vi "Auto Intake Mode.vi"(7 "Intake Angle":dbl, 11 "Intake Commands Cluster":T2={"Intake Commands"=enum."Load", "Intake Mode"=enum."Auto", "Override IR"=FALSE, "Angle Target"=0.0}) -> (0 "Intake States":T1, 1 "Limit with Encoders?":bool, 2 "Roller Power":dbl, 3 "Angle Power":dbl, 4 "Target Height":dbl, 5 "Encoder Position":dbl, 6 "Rollers Active?":bool)   [LabVIEW 2015]
uses:
  Common Code/Intake Commands Cluster.ctl
  Common Code/Intake Commands.ctl
  Common Code/Intake Mode.ctl
  Common Code/Intake States.ctl
  Common Code/Change Detect Int.vi
  Common Code/Change Detect Double.vi
  Robot Global Data.vi
  <vilib>/addons/control/pid/pid.llb/PID (DBL).vi
  <vilib>/addons/control/pid/NI_PID_pid.lvlib
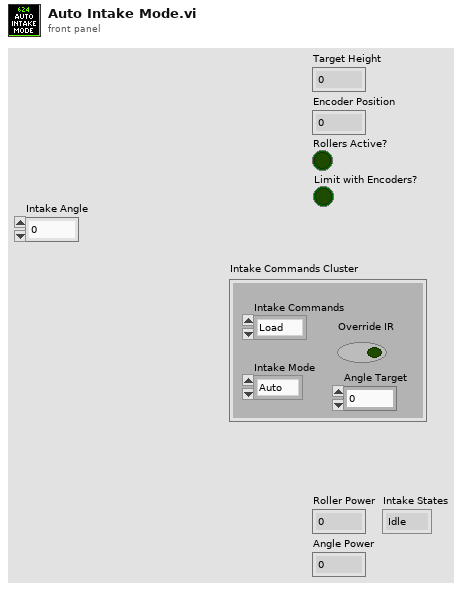
[diagram p1: front panel]
types:
  T1 = typedef "Intake States.ctl" = enum16{"Idle", "Set roller speed", "Move to angle", "Go Hard or Go Home", "Ball Settle"}
  T2 = typedef "Intake Commands Cluster.ctl" = cluster{"Intake Commands":T3, "Intake Mode":T4, "Override IR":bool, "Angle Target":dbl}
  T3 = typedef "Intake Commands.ctl" = enum16{"Settle Ball", "Unload", "Load", "Pull up", "Drop low", "Idle", "Lift Half", "Go To Angle"}
  T4 = typedef "Intake Mode.ctl" = enum16{"Safe", "Auto", "Manual"}
  T5 = typedef "Dashboard Control Data.ctl" = cluster{"Shooter Presets":T6, "Encoder Control":T8, "Steer PID output":cluster{"output high":dbl, "output low":dbl}, " Steer PID gains":cluster{"proportional gain (Kc)":dbl, "integral time (Ti, min)":dbl, "derivative time (Td, min)":dbl}, "Drivetrain Settings":T9, "Vision Packet":T10, "Dashboard Drivetrain Command":T11, "Info/Command Cluster":T13, "Ball Vision Packet":T14, "Intake Presets":T16, "Intake Encoder Control":T18, "Climb Presets":T19, "Goal Output Range":cluster{"output high":dbl, "output low":dbl}, "Enabled Systems":T20, "Auton Presets":T21, "Pressure M":dbl, "Pressure B":dbl, "Vision Timeout":dbl, "Auto-Shift":T22}
  T6 = typedef "Shooter Presets.ctl" = cluster{"Batter Shot":T7, "Deep Middle":T7, "Manual Shot":T7, "Left Ticks Per Rotation":dbl, "Right Ticks Per Rotation":dbl, "Low Bar Shot":T7, "Shooter RPM Tolerance":dbl, "Trigger Power":dbl, "Fire from Load Delay":i32, "Max Angle":dbl, "Min Angle":dbl, "Angle PID gains":cluster{"P":dbl, "I":dbl, "D":dbl}, "Angle Output":cluster{"output high":dbl, "output low":dbl}, "Shooter Angle Tolerance":dbl, "Vision Shoot x^2":dbl, "Vision Shoot x":dbl, "Feed Forward Max Accel":dbl, "Feed Forward Kv":dbl, "Backwards Trigger":dbl, "Shot Finish Delay (ms)":dbl, "Angle Max Current":dbl, "Angle Current Trip Time":dbl, "Intake Angle":dbl, "Vision Shoot c":dbl, "Reset?":bool, "Button Release Delay":dbl, "Angle Pot x":dbl, "Angle Pot c":dbl, "Ignore Angle?":bool, "Max RPM":dbl, "Safty Frist Angle":dbl, "Intake Danger Height":dbl, "Angle Pot B":i32, "Angle Pot M":dbl, "FF Finish RPM":dbl, "RPM PID Right":cluster{"P":dbl, "I":dbl, "D":dbl, "FF":dbl}, "RPM PID Left":cluster{"P":dbl, "I":dbl, "D":dbl, "FF":dbl}, "Backwards RPM":dbl, "Vision RPM":dbl, "Run Wheels Backward Delay":u32, "Cleat Shot":T7}
  T7 = typedef "Shot Presets.ctl" = cluster{"L":dbl, "R":dbl, "A":dbl}
  T8 = typedef "Encoder Control.ctl" = cluster{"Right Tick Constant":dbl, "Left Tick Constant":dbl, "Reset?":bool, "Y Dist":cluster{"PID gains":cluster{"proportional gain (Kc)":dbl, "integral time (Ti, min)":dbl, "derivative time (Td, min)":dbl}}, "Y Stop Thresh":dbl, "Y Stop Speed":dbl}
  T9 = typedef "Drivetrain Settings.ctl" = cluster{"Gyro Tolerance":dbl, "Throttle Ramp (ms)":dbl, "Kv":dbl, "Ka":dbl, "Feed Forward P":dbl, "Feed Forward D":dbl, "Goal Vision PID gains":cluster{"proportional gain (Kc)":dbl, "integral time (Ti, min)":dbl, "derivative time (Td, min)":dbl}, "Goal Detection Window":dbl, "Creep Rate":dbl, "Vision Throttle Threshold":dbl, "Min Turn Output":dbl, "Left Batter Angle":dbl, "Right Batter Angle":dbl}
  T10 = typedef "Goal Vision Packet.ctl" = cluster{"Distance":dbl, "Center X":dbl, "Center Y":dbl, "Found Target?":bool, "Robot Center":dbl, "Angle":dbl}
  T11 = typedef "Dashboard Drivetrain Command.ctl" = cluster{"Drivetrain Vision":T12}
  T12 = typedef "Drivetrain Vision.ctl" = cluster{"Goal Window":dbl, "Ball Window":dbl}
  T13 = typedef "Ball Tracking Command Cluster.ctl" = cluster{"Distance to Ball":dbl, "Desired Angle":dbl, "Command":enum16{"Turn to Ball", "Turn to Angle", "Get Distance"}, "Pixels from Center":dbl}
  T14 = typedef "Ball Vision Packet.ctl" = cluster{"Ball Detected?":bool, "Distance to Ball":dbl, "Desired Angle":dbl, "Pixels from Center":dbl, "Tracking mode":T15}
  T15 = typedef "Tracking Mode.ctl" = enum16{"Turn to Ball", "Turn to Angle"}
  T16 = typedef "Intake Presets.ctl" = cluster{"Intake Speed":dbl, "Outake Speed":dbl, "Low Height":dbl, "Half Height":dbl, "High Idle Height":dbl, "Angle Speed":dbl, "Angle Tolerance":dbl, "Encoder Scale":dbl, "Load Height":dbl, "Output Range":T17, "Rotation Power Max/Min":dbl, "MaxCurrent":dbl, "Intake Trip Time":dbl, "Idle Height":dbl, "Max Height":dbl, "Reset Encoders?":bool, "PID gains":cluster{"proportional gain (Kc)":dbl, "integral time (Ti, min)":dbl, "derivative time (Td, min)":dbl}, "Intake Stop Delay":u32, "Settle Time":dbl, "Settle Wait Time":dbl, "Pull Up Delay":dbl}
  T17 = typedef "Drivetrain Output Range.ctl" = cluster{"output high":dbl, "output low":dbl}
  T18 = typedef "IntakeEcoderControl.ctl" = cluster{"Arm Tick Constant":dbl, "Reset?":bool, "Y Dist":cluster{"PID gains":cluster{"proportional gain (Kc)":dbl, "integral time (Ti, min)":dbl, "derivative time (Td, min)":dbl}}, "Y Stop Thresh":dbl, "Y Stop Speed":dbl}
  T19 = typedef "Climb Presets.ctl" = cluster{"Pull Power":dbl, "Extend Power":dbl}
  T20 = typedef "Enabled Systems.ctl" = cluster{"Shoot":bool, "Intake":bool, "DT":bool, "Gyro":bool, "100ms":bool, "US":bool}
  T21 = typedef "Autonomous Presets.ctl" = cluster{"Pitch Limit":dbl, "Roll Limit":dbl, "Start Position":dbl, "Cross Position":dbl}
  T22 = typedef "Auto Shift Cluster.ctl" = cluster{"Delay":dbl, "Speed Thresh":dbl, "Upshift Accel":dbl, "Upshift Throttle":dbl, "Upshift Throttle Accel":dbl, "Downshift Throttle":dbl, "Downshift Throttle Accel":dbl}
  T23 = cluster{"proportional gain (Kc)":dbl, "integral time (Ti, min)":dbl, "derivative time (Td, min)":dbl}
  T24 = typedef "Shooter State Cluster.ctl" = cluster{"State":T25, "Left RPM":dbl, "Right RPM":dbl, "Shooter Ready?":bool, "Ball Loaded?":bool, "Current Angle":dbl, "Angle Motor Output":dbl, "Trigger Output":dbl, "Angle Ready?":bool, "RPM Ready?":bool, "Vision Ready?":bool, "Ball Loaded?":bool, "Mode":T26, "Shot Type":T27, "Pot Height":dbl, "Current Tripped Forward?":bool, "Current Tripped Backward?":bool, "Right Servo":i32, "Left Servo":i32, "IR Override":bool, "Intake Danger?":bool, "Intake Angle Ready?":bool}
  T25 = typedef "Shooter State.ctl" = enum16{"Idle", "Settle Ball", "Warmup", "Shooter Ready", "Shoot"}
  T26 = typedef "Shoot Modes Enum.ctl" = enum16{"Manual", "Safe", "Auto"}
  T27 = typedef "Shot Type.ctl" = enum16{"Batter Shot", "Corner Shot", "Cleat Shot", "Vision Shot", "Deep Middle Shot"}
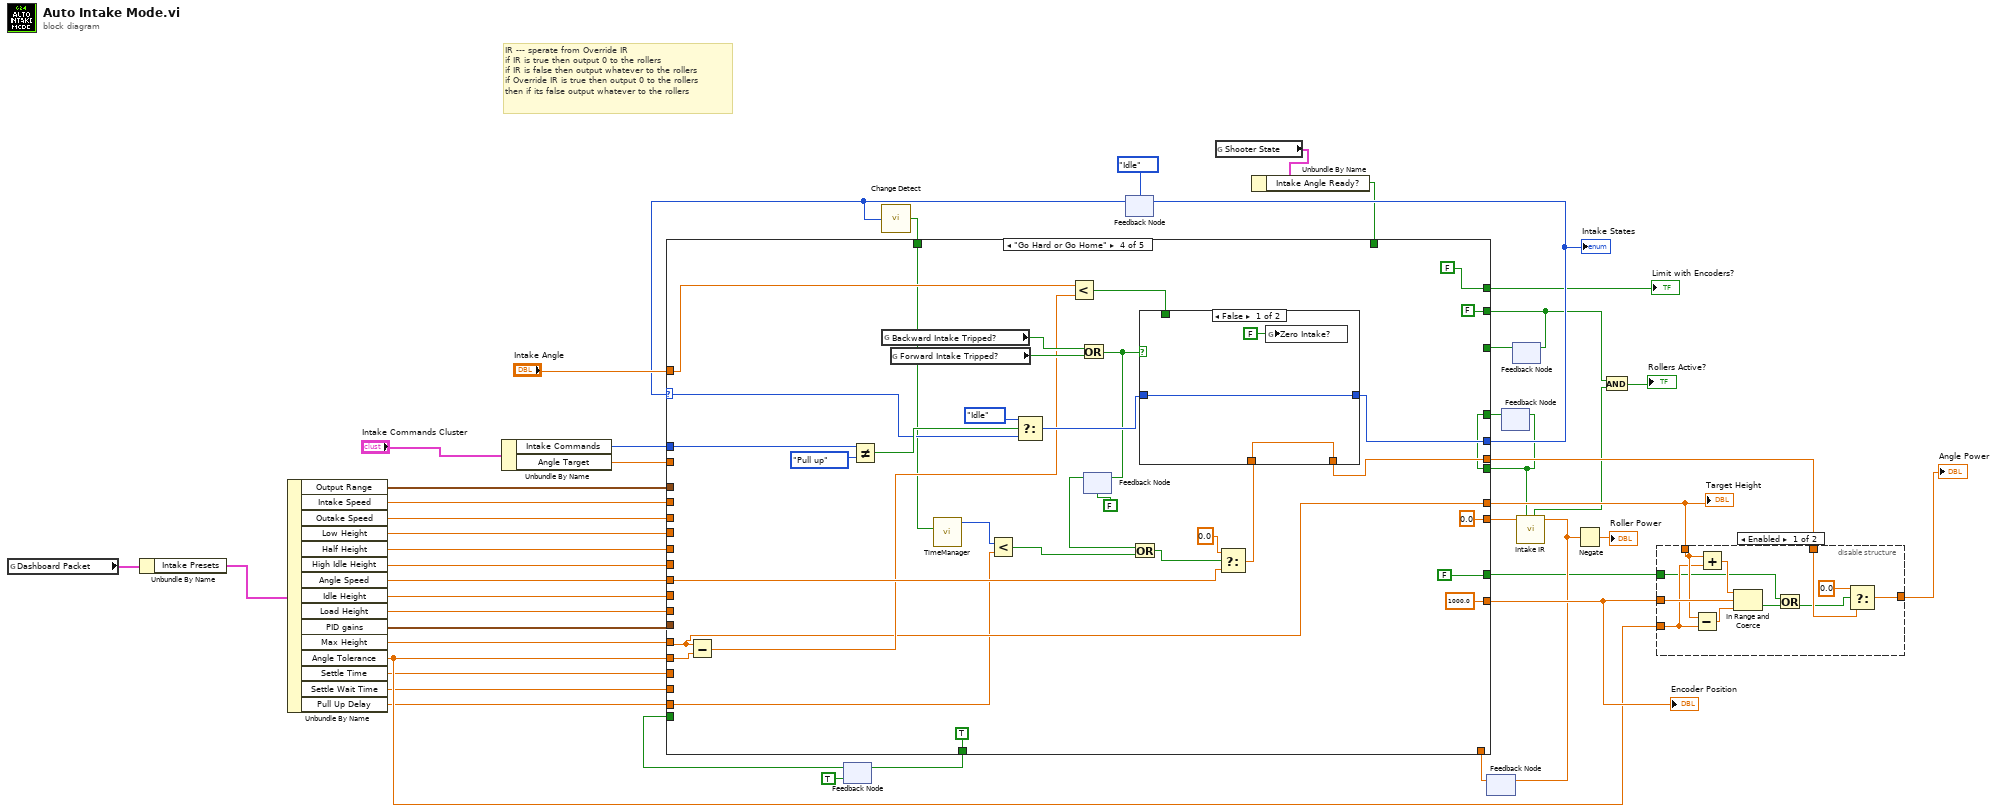
[diagram p0: block diagram]
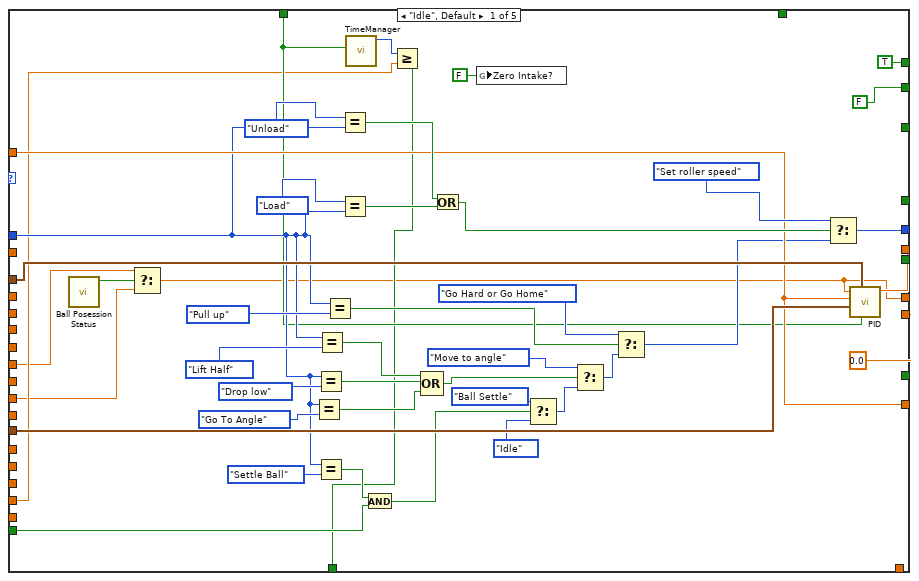
[diagram p3: hidden frame]
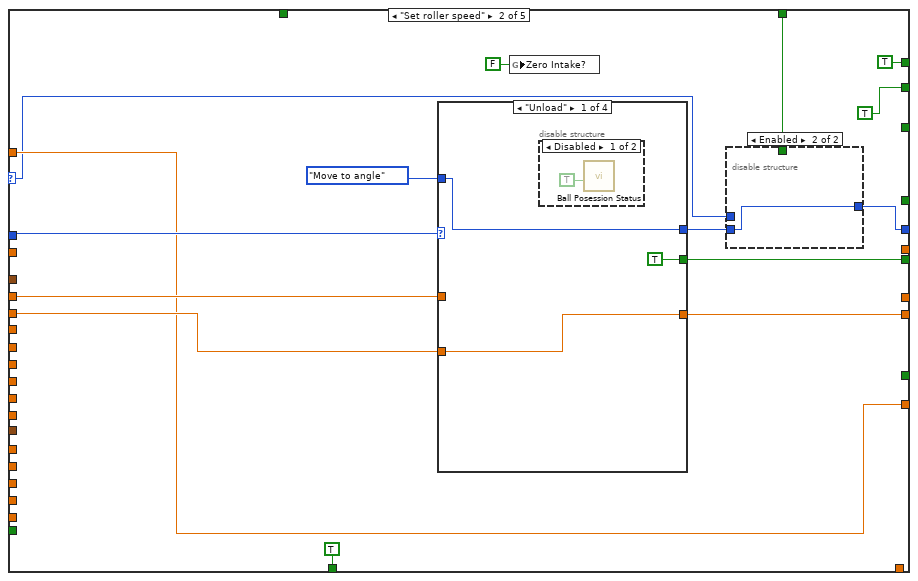
[diagram p4: hidden frame]
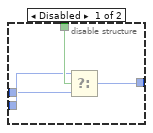
[diagram p5: hidden frame]
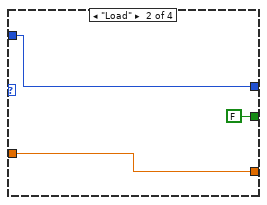
[diagram p7: hidden frame]
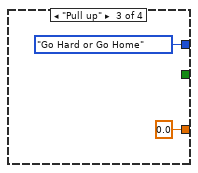
[diagram p8: hidden frame]
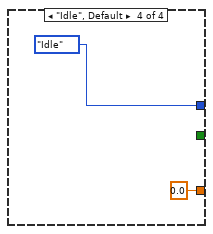
[diagram p9: hidden frame]
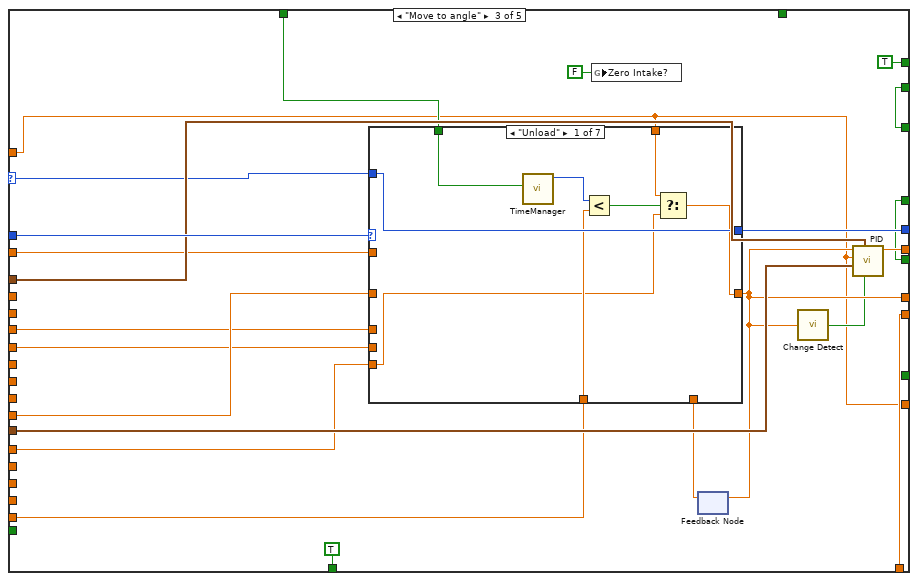
[diagram p10: hidden frame]
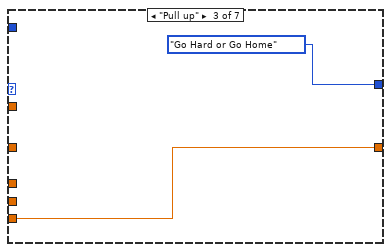
[diagram p12: hidden frame]
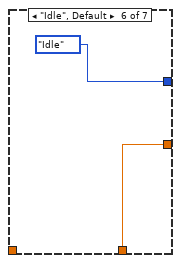
[diagram p15: hidden frame]
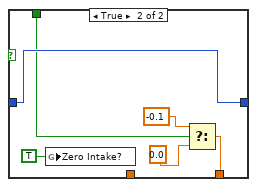
[diagram p17: hidden frame]
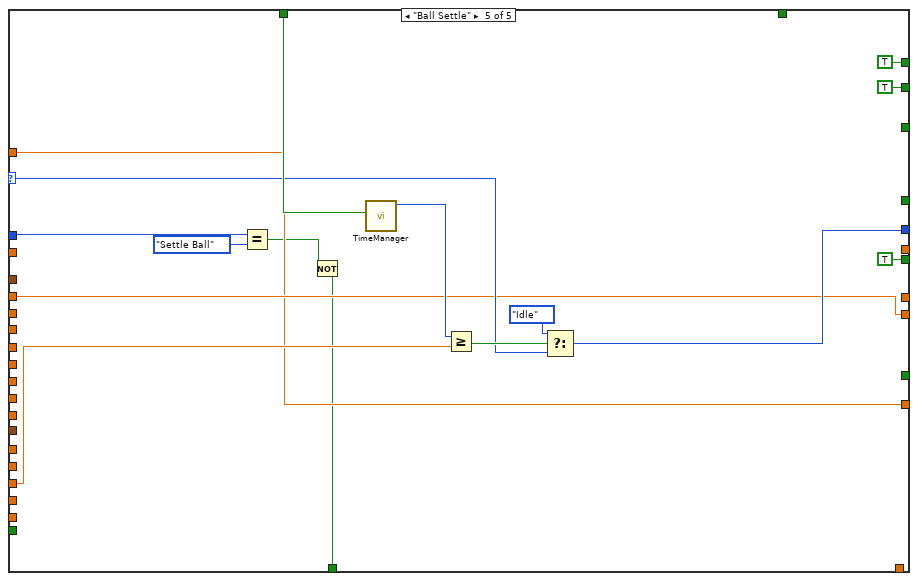
[diagram p18: hidden frame]
diagram:
  # "IR --- sperate from Override IR \nif IR is true then output 0 to the rollers\nif IR is false then output whatever to the rollers\nif Override IR is true then output 0 to the rollers\nthen if its false output whatever to the rollers"
  n1 = global read "Robot Global Data.vi" "Dashboard Packet"() -> (w30:T5)
  n2 = Unbundle By Name(w30) -> ("Intake Presets"=w31:T16)
  n3 = Unbundle By Name(w31) -> ("Output Range"=w41:T17, "Intake Speed"=w40:dbl, "Outake Speed"=w39:dbl, "Low Height"=w38:dbl, "Half Height"=w37:dbl, "High Idle Height"=w36:dbl, "Angle Speed"=w35:dbl, "Idle Height"=w34:dbl, "Load Height"=w33:dbl, "PID gains"=w32:T23, "Max Height"=w29:dbl, "Angle Tolerance"=w7:dbl, "Settle Time"=w6:dbl, "Settle Wait Time"=w2:dbl, "Pull Up Delay"=w1:dbl)
  n4 = Unbundle By Name("Intake Commands Cluster") -> ("Intake Commands"=w44:T3, "Angle Target"=w10:dbl)
  n5 = feedback #1(TRUE) -> (w4:bool)
  n6 = feedback #2(Intake_States."Idle") -> (w24:T1)
  n7 = call-poly "Change Detect.vi"("In"=w24) -> ("Changed?"=w23:bool)
  n8 = global read "Robot Global Data.vi" "Shooter State"() -> (w9:T24)
  n9 = Unbundle By Name(w9) -> ("Intake Angle Ready?"=w8:bool)
  n10 = feedback #3() -> (w42:dbl)  [unwired: 1 in]
  n11 = feedback #4() -> (w12:bool)  [unwired: 1 in]
  n12 = feedback #5() -> (w11:bool)  [unwired: 1 in]
  n13 = case shown="\"Go Hard or Go Home\"" w24 {
    selector: w24 -> [_ w93 w134 w187 w218]
    tunnel: w44 -> [w62 w105 w144 w190 w216]
    tunnel: [w83 w92 w135 w192 w214] -> w43
    tunnel: w41 -> [w74 _ w137 _ _]
    tunnel: w39 -> [_ w102 _ _ _]
    tunnel: w36 -> [w47 _ _ _ _]
    tunnel: w40 -> [_ w103 _ _ w212]
    tunnel: w37 -> [_ _ w141 _ _]
    tunnel: w35 -> [_ _ _ w181 _]
    tunnel: w38 -> [_ _ w140 _ _]
    tunnel: [0.0 ("Intake Speed") w99 w143 0.0 ("Speeeeeeed") w212] -> w20
    tunnel: w42 -> [_ _ w143 _ _]
    tunnel: w33 -> [_ _ w142 _ _]
    tunnel: [w73 _ w139 w183 _] -> w21
    tunnel: "Intake Angle" -> [w71 w100 w122 w177 w211]
    tunnel: w32 -> [w75 _ w138 _ _]
    tunnel: w34 -> [w49 _ _ _ _]
    tunnel: [w48 _ w133 w172 _] -> w27
    tunnel: [w71 w100 w122 1000.0 ("Intake Angle") w211] -> w28
    tunnel: [FALSE TRUE w128 FALSE TRUE] -> w17
    tunnel: w29 -> [_ _ w125 w172 _]
    tunnel: w23 -> [w54 _ w124 w170 w222]
    tunnel: [_ w98 w130 w182 TRUE] -> w13
    tunnel: [_ _ _ FALSE _] -> w15
    tunnel: [TRUE TRUE TRUE FALSE TRUE] -> w14
    tunnel: w12 -> [_ _ w130 w182 _]
    tunnel: w11 -> [_ _ w128 _ _]
    tunnel: w10 -> [_ _ w127 _ _]
    tunnel: w8 -> [_ w95 _ _ _]
    tunnel: w7 -> [_ _ _ w176 _]
    tunnel: w6 -> [_ _ _ _ w221]
    tunnel: [w52 TRUE TRUE TRUE w207] -> w5
    tunnel: w4 -> [w59 _ _ _ _]
    tunnel: w2 -> [w51 _ _ _ _]
    tunnel: w1 -> [_ _ w123 w168 _]
    frame "Idle", Default {
      n14 = call "Ball Posession Status.vi"() -> ("Ball Posessed?"=w50:bool)  [unwired: 11 in]
      n15 = Select(t=w47, s=w50, f=w49) -> (s? t:f=w48:dbl)
      n16 = Equal?(x=w62, y=Intake_Commands."Go To Angle" ("Intake Commands")) -> (x = y?=w63:bool)
      n17 = Equal?(x=w62, y=Intake_Commands."Drop low" ("Intake Commands")) -> (x = y?=w84:bool)
      n18 = Equal?(x=w62, y=Intake_Commands."Settle Ball") -> (x = y?=w60:bool)
      n19 = Equal?(x=w62, y=Intake_Commands."Lift Half" ("Intake Commands")) -> (x = y?=w85:bool)
      n20 = Equal?(x=w62, y=Intake_Commands."Pull up" ("Intake Commands")) -> (x = y?=w69:bool)
      n21 = Equal?(x=Intake_Commands."Unload" ("Intake Commands"), y=w62) -> (x = y?=w79:bool)
      n22 = Equal?(x=Intake_Commands."Load" ("Intake Commands"), y=w62) -> (x = y?=w78:bool)
      n23 = call "TimeManager.vi"("Reset?"=w54) -> ("Time Since Reset"=w53:u32)  [unwired: 9 in, 1 out]
      n24 = And(x=w60, y=w59) -> (x .and. y?=w56:bool)
      n25 = Greater Or Equal?(x=w53, y=w51) -> (x >= y?=w52:bool)
      n26 = Compound Arithmetic op=OR(w85, w84, w63) -> (w88:bool)
      n27 = Or(x=w79, y=w78) -> (x .or. y?=w77:bool)
      n28 = global write "Robot Global Data.vi" "Zero Intake?"(FALSE ("Zero Intake?")) -> ()
      n29 = Select(t=Intake_States."Ball Settle", s=w56, f=Intake_States."Idle") -> (s? t:f=w58:T1)
      n30 = Select(t=Intake_States."Move to angle", s=w88, f=w58) -> (s? t:f=w70:T1)
      n31 = Select(t=Intake_States."Go Hard or Go Home", s=w69, f=w70) -> (s? t:f=w67:T1)
      n32 = Select(t=Intake_States."Set roller speed", s=w77, f=w67) -> (s? t:f=w83:T1)
      n33 = call-poly <vilib>:"PID.vi"("reinitialize? (F)"=w54, "output range"=w74, "PID gains"=w75, "process variable"=w71, "setpoint"=w48) -> ("output"=w73:dbl)  [unwired: 5 in, 1 out]
    }
    frame "Set roller speed" {
      n34 = case shown="\"Unload\"" w105 {
        tunnel: Intake_States."Move to angle" -> [w113 w117 _ _]
        tunnel: [w113 w117 Intake_States."Go Hard or Go Home" Intake_States."Idle"] -> w94
        tunnel: w103 -> [_ w116 _ _]
        tunnel: [w112 w116 0.0 ("Intake Speed") 0.0 ("Intake Speed")] -> w99
        tunnel: w102 -> [w112 _ _ _]
        tunnel: [TRUE FALSE _ _] -> w98
        frame "Unload" {
          n35 = disable-structure shown="Disabled" {
            frame Disabled {
              n36 = call "Ball Posession Status.vi"("Logical Exit?"=TRUE) -> ()  [unwired: 10 in, 1 out]
            }
            frame Enabled {
            }
          }
        }
        frame "Load" {
        }
        frame "Pull up" {
        }
        frame "Idle", Default {
        }
      }
      n37 = global write "Robot Global Data.vi" "Zero Intake?"(FALSE ("Zero Intake?")) -> ()
      n38 = disable-structure shown="Enabled" {
        disable-tunnel: w95 -> [w109 _]
        disable-tunnel: w94 -> [w108 w110]
        disable-tunnel: w93 -> [w107 _]
        disable-tunnel: [w106 w110] -> w92
        frame Disabled {
          n39 = Select(t=w108, s=w109, f=w107) -> (s? t:f=w106:T1)
        }
        frame Enabled {
        }
      }
    }
    frame "Move to angle" {
      n40 = global write "Robot Global Data.vi" "Zero Intake?"(FALSE ("Zero Intake?")) -> ()
      n41 = feedback #6() -> (w136:dbl)  [unwired: 1 in]
      n42 = case shown="\"Unload\"" w144 {
        tunnel: w142 -> [_ w154 _ _ _ _ _]
        tunnel: [w145 w154 w156 w158 w159 w162 w164] -> w133
        tunnel: w141 -> [_ _ _ _ _ _ w164]
        tunnel: w140 -> [_ _ _ w158 _ _ _]
        tunnel: w125 -> [w146 _ w156 _ _ _ _]
        tunnel: w136 -> [_ _ _ _ _ w162 _]
        tunnel: [w152 w153 Intake_States."Go Hard or Go Home" w157 w160 Intake_States."Idle" w163] -> w135
        tunnel: w134 -> [w152 w153 _ w157 w160 _ w163]
        tunnel: w127 -> [_ _ _ _ w159 _ _]
        tunnel: w124 -> [w150 _ _ _ _ _ _]
        tunnel: w123 -> [w149 _ _ _ _ _ _]
        tunnel: w122 -> [w147 _ _ _ _ _ _]
        frame "Unload" {
          n43 = call "TimeManager.vi"("Reset?"=w150) -> ("Time Since Reset"=w151:u32)  [unwired: 9 in, 1 out]
          n44 = Less?(x=w151, y=w149) -> (x < y?=w148:bool)
          n45 = Select(t=w147, s=w148, f=w146) -> (s? t:f=w145:dbl)
        }
        frame "Load" {
        }
        frame "Pull up" {
        }
        frame "Drop low" {
        }
        frame "Go To Angle" {
        }
        frame "Idle", Default {
        }
        frame "Lift Half" {
        }
      }
      n46 = feedback-in #6(w133) -> ()
      n47 = call-poly "Change Detect.vi"("In"=w133) -> ("Changed?"=w132:bool)
      n48 = call-poly <vilib>:"PID.vi"("reinitialize? (F)"=w132, "output range"=w137, "PID gains"=w138, "process variable"=w122, "setpoint"=w133) -> ("output"=w139:dbl)  [unwired: 5 in, 1 out]
    }
    frame "Go Hard or Go Home" {
      n49 = Subtract(x=w172, y=w176) -> (x-y=w175:dbl)
      n50 = Not Equal?(x=w190, y=Intake_Commands."Pull up") -> (x != y?=w189:bool)
      n51 = global read "Robot Global Data.vi" "Backward Intake Tripped?"() -> (w194:bool)
      n52 = global read "Robot Global Data.vi" "Forward Intake Tripped?"() -> (w193:bool)
      n53 = call "TimeManager.vi"("Reset?"=w170) -> ("Time Since Reset"=w169:u32)  [unwired: 9 in, 1 out]
      n54 = Less?(x=w169, y=w168) -> (x < y?=w166:bool)
      n55 = Select(t=Intake_States."Idle", s=w189, f=w187) -> (s? t:f=w186:T1)
      n56 = Less?(x=w177, y=w175) -> (x < y?=w173:bool)
      n57 = Or(x=w194, y=w193) -> (x .or. y?=w174:bool)
      n58 = feedback-in #7(w174) -> ()
      n59 = feedback #7(FALSE) -> (w167:bool)
      n60 = Or(x=w167, y=w166) -> (x .or. y?=w165:bool)
      n61 = Select(t=0.0, s=w165, f=w181) -> (s? t:f=w180:dbl)
      n62 = case shown="False" w174 {
        tunnel: [w198 w205] -> w192
        tunnel: w186 -> [w198 w205]
        tunnel: w180 -> [w200 _]
        tunnel: [w200 w203] -> w183
        tunnel: w173 -> [_ w201]
        frame False {
          n63 = global write "Robot Global Data.vi" "Zero Intake?"(FALSE ("Zero Intake?")) -> ()
        }
        frame True {
          n64 = global write "Robot Global Data.vi" "Zero Intake?"(TRUE ("Zero Intake?")) -> ()
          n65 = Select(t=-0.1, s=w201, f=0.0 ("Angle Speed")) -> (s? t:f=w203:dbl)
        }
      }
    }
    frame "Ball Settle" {
      n66 = Equal?(x=w216, y=Intake_Commands."Settle Ball") -> (x = y?=w208:bool)
      n67 = Not(x=w208) -> (.not. x?=w207:bool)
      n68 = call "TimeManager.vi"("Reset?"=w222) -> ("Time Since Reset"=w220:u32)  [unwired: 9 in, 1 out]
      n69 = Greater Or Equal?(x=w220, y=w221) -> (x >= y?=w219:bool)
      n70 = Select(t=Intake_States."Idle", s=w219, f=w218) -> (s? t:f=w214:T1)
    }
  }
  "Intake States" <- w43
  "Target Height" <- w27
  "Encoder Position" <- w28
  "Limit with Encoders?" <- w14
  n71 = feedback-in #1(w5) -> ()
  n72 = feedback-in #2(w43) -> ()
  n73 = feedback-in #4(w13) -> ()
  n74 = feedback-in #5(w17) -> ()
  n75 = call "Intake IR.vi"("Unload?"=w13, "Speed"=w20) -> ("Speeeeeeed"=w19:dbl, "Rollers Enabled?"=w18:bool)  [unwired: 8 in]
  n76 = feedback-in #3(w19) -> ()
  n77 = Negate(x=w19) -> (-x=→"Roller Power":dbl)
  n78 = And(x=w17, y=w18) -> (x .and. y?=→"Rollers Active?":bool)
  n79 = disable-structure shown="Enabled" {
    disable-tunnel: w28 -> [w233 _]
    disable-tunnel: w27 -> [w232 _]
    disable-tunnel: w7 -> [w231 _]
    disable-tunnel: [w226 w234] -> w26
    disable-tunnel: w21 -> [w225 w234]
    disable-tunnel: w15 -> [w223 _]
    frame Enabled {
      n80 = Subtract(x=w232, y=w231) -> (x-y=w230:dbl)
      n81 = Add(x=w232, y=w231) -> (x+y=w229:dbl)
      n82 = In Range and Coerce(upper limit=w229, x=w233, lower limit=w230) -> (In Range?=w228:bool)  [unwired: 1 out]
      n83 = Or(x=w223, y=w228) -> (x .or. y?=w224:bool)
      n84 = Select(t=0.0, s=w224, f=w225) -> (s? t:f=w226:dbl)
    }
    frame Disabled {
    }
  }
  "Angle Power" <- w26
